vi "Advance Folder Operation.vi"(0 "VISA resource name":refnum<visa-resource-name>, 1 "New File Name":string, 5 "Folder Operation (3: Query Path Type)":i32(ring)=3 items=["Rename File", "Remove File", "Remove Folder", "Query Path Type", "Create New Folder", "List Folder Files"], 7 "File Name":string, 9 "Path (/usb1/)":string="/usb1/", 11 "error in (no error)":errorcluster) -> (3 "Folder File List":string[](array[string]), 4 "VISA resource name out":refnum<visa-resource-name>, 6 "Directory":bool, 8 "File":bool, 10 "Path":string, 15 "error out":errorcluster)   [LabVIEW 2019, in "Keithley 2600 Series.lvlib"]
doc: "Advance operations for the folder and files."
uses:
  Keithley 2600 Series.lvlib
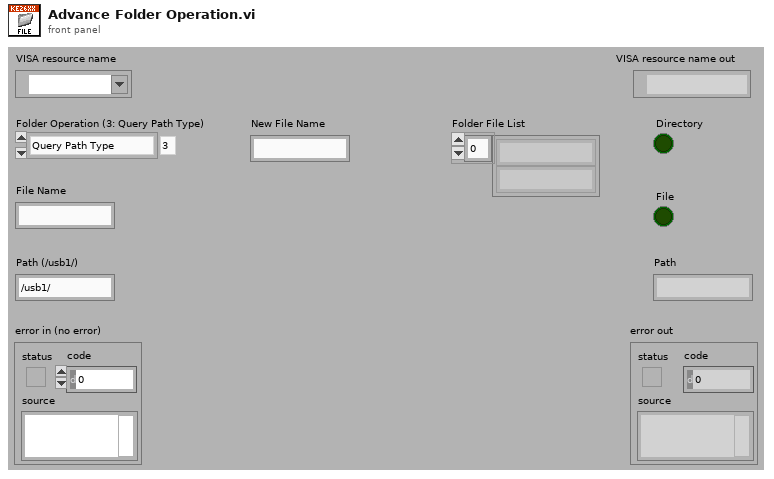
[diagram p1: front panel]
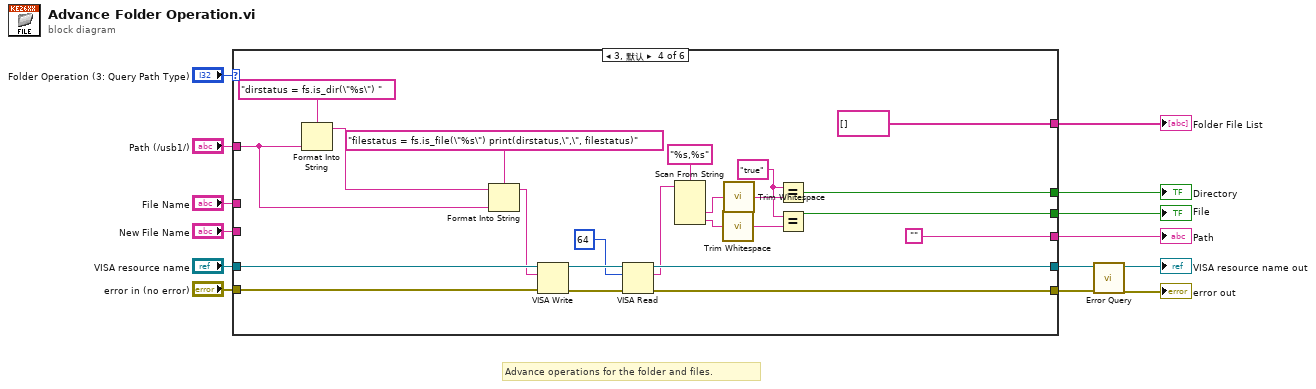
[diagram p0: block diagram]
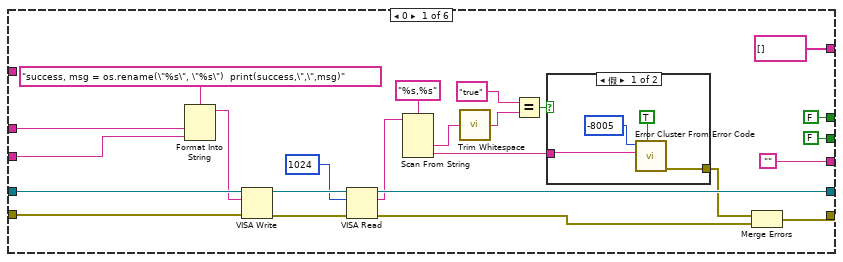
[diagram p2: hidden frame]
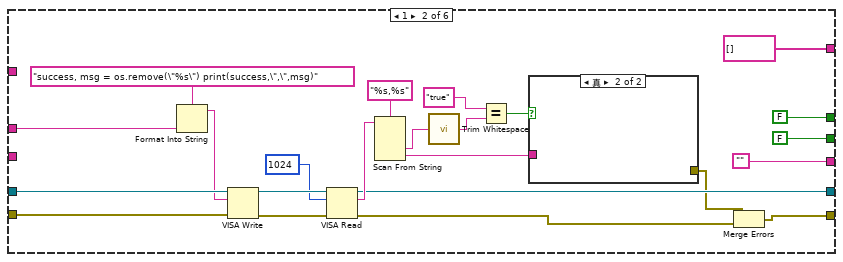
[diagram p4: hidden frame]
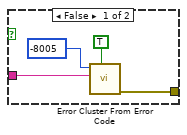
[diagram p5: hidden frame]
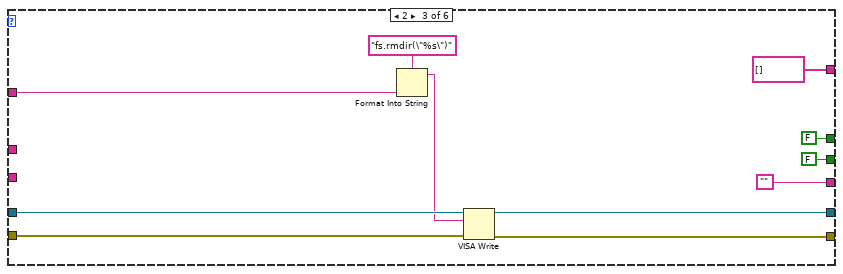
[diagram p6: hidden frame]
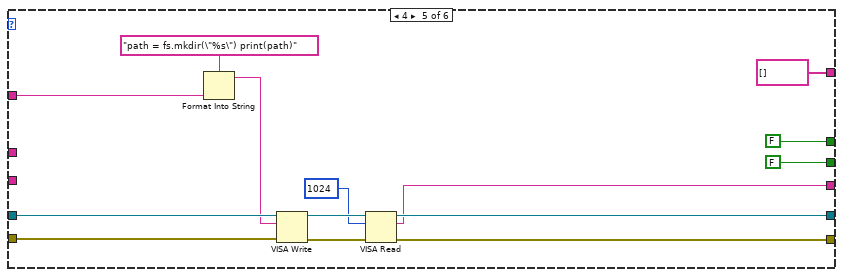
[diagram p7: hidden frame]
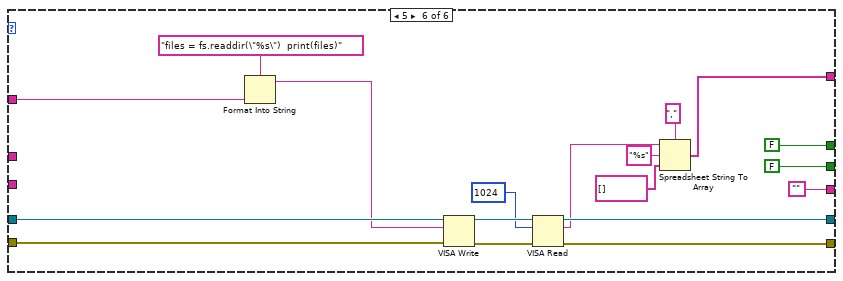
[diagram p8: hidden frame]
diagram:
  # "Advance operations for the folder and files."
  n1 = case shown="3, 默认" "Folder Operation (3: Query Path Type)" {
    tunnel: "VISA resource name" -> [w34 w53 w78 w101 w112 w130]
    tunnel: "error in (no error)" -> [w33 w52 w77 w100 w111 w129]
    tunnel: [w28 w50 w75 w97 w109 w127] -> w4
    tunnel: [w19 w43 w74 w96 w108 w126] -> w3
    tunnel: "Path (/usb1/)" -> [_ _ w79 w95 w113 w131]
    tunnel: "File Name" -> [w32 w64 _ _ _ _]
    tunnel: "New File Name" -> [w31 _ _ _ _ _]
    tunnel: ["" "" "" "" w107 ""] -> w6
    tunnel: [string[] [] string[] [] string[] [] string[] [] string[] [] w122] -> w5
    tunnel: [FALSE FALSE FALSE w82 FALSE FALSE] -> w2
    tunnel: [FALSE FALSE FALSE w81 FALSE FALSE] -> w1
    frame 0 {
      n2 = Format Into String(format string="success, msg = os.rename(\"%s\", \"%s\")  print(success,\",\",msg)", w32, w31) -> (resulting string=w30:string)  [unwired: 2 in, 1 out]
      n3 = VISA Write(VISA resource name=w34, write buffer=w30, error in (no error)=w33) -> (VISA resource name out=w37:refnum<visa-resource-name>, error out=w36:errorcluster)  [unwired: 1 out]
      n4 = VISA Read(VISA resource name=w37, byte count=u32 1024, error in (no error)=w36) -> (VISA resource name out=w28:refnum<visa-resource-name>, read buffer=w27:string, error out=w17:errorcluster)  [unwired: 1 out]
      n5 = Scan From String(format string="%s,%s", input string=w27) -> (output 1=w26:string, output 2=w22:string)  [unwired: 4 in, 3 out]
      n6 = call <vilib>:"Trim Whitespace.vi"("string"=w26) -> ("trimmed string"=w25:string)  [unwired: 1 in]
      n7 = Equal?(x="true", y=w25) -> (x = y?=w23:bool)
      n8 = case shown="假" w23 {
        tunnel: w22 -> [w42 _]
        tunnel: [w40 _] -> w18
        frame False {
          n9 = call <vilib>:"Error Cluster From Error Code.vi"("show call chain? (False)"=TRUE, "error message (\"\")"=w42, "error code (0)"=-8005) -> ("error out"=w40:errorcluster)  [unwired: 6 in]
        }
        frame True {
        }
      }
      n10 = Merge Errors(w18, w17) -> (w19:errorcluster)
    }
    frame 1 {
      n11 = Format Into String(format string="success, msg = os.remove(\"%s\") print(success,\",\",msg)", w64) -> (resulting string=w51:string)  [unwired: 2 in, 1 out]
      n12 = VISA Write(VISA resource name=w53, write buffer=w51, error in (no error)=w52) -> (VISA resource name out=w63:refnum<visa-resource-name>, error out=w62:errorcluster)  [unwired: 1 out]
      n13 = VISA Read(VISA resource name=w63, byte count=u32 1024, error in (no error)=w62) -> (VISA resource name out=w50:refnum<visa-resource-name>, read buffer=w59:string, error out=w46:errorcluster)  [unwired: 1 out]
      n14 = Scan From String(format string="%s,%s", input string=w59) -> (output 1=w58:string, output 2=w54:string)  [unwired: 4 in, 3 out]
      n15 = call <vilib>:"Trim Whitespace.vi"("string"=w58) -> ("trimmed string"=w57:string)  [unwired: 1 in]
      n16 = Equal?(x="true", y=w57) -> (x = y?=w55:bool)
      n17 = case shown="真" w55 {
        tunnel: w54 -> [w69 _]
        tunnel: [w67 _] -> w47
        frame False {
          n18 = call <vilib>:"Error Cluster From Error Code.vi"("show call chain? (False)"=TRUE, "error message (\"\")"=w69, "error code (0)"=-8005) -> ("error out"=w67:errorcluster)  [unwired: 6 in]
        }
        frame True {
        }
      }
      n19 = Merge Errors(w47, w46) -> (w43:errorcluster)
    }
    frame 2 {
      n20 = Format Into String(format string="fs.rmdir(\"%s\")", w79) -> (resulting string=w76:string)  [unwired: 2 in, 1 out]
      n21 = VISA Write(VISA resource name=w78, write buffer=w76, error in (no error)=w77) -> (VISA resource name out=w75:refnum<visa-resource-name>, error out=w74:errorcluster)  [unwired: 1 out]
    }
    frame 3, Default {
      w85 = "true"
      n22 = Format Into String(format string="dirstatus = fs.is_dir(\"%s\") ", w95) -> (resulting string=w94:string)  [unwired: 2 in, 1 out]
      n23 = Format Into String(format string="filestatus = fs.is_file(\"%s\") print(dirstatus,\",\", filestatus)", initial string=w94, w95) -> (resulting string=w93:string)  [unwired: 1 in, 1 out]
      n24 = VISA Write(VISA resource name=w101, write buffer=w93, error in (no error)=w100) -> (VISA resource name out=w99:refnum<visa-resource-name>, error out=w98:errorcluster)  [unwired: 1 out]
      n25 = VISA Read(VISA resource name=w99, byte count=u32 64, error in (no error)=w98) -> (VISA resource name out=w97:refnum<visa-resource-name>, read buffer=w91:string, error out=w96:errorcluster)  [unwired: 1 out]
      n26 = Scan From String(format string="%s,%s", input string=w91) -> (output 1=w89:string, output 2=w88:string)  [unwired: 4 in, 3 out]
      n27 = call <vilib>:"Trim Whitespace.vi"("string"=w88) -> ("trimmed string"=w86:string)  [unwired: 1 in]
      n28 = call <vilib>:"Trim Whitespace.vi"("string"=w89) -> ("trimmed string"=w87:string)  [unwired: 1 in]
      n29 = Equal?(x=w85, y=w87) -> (x = y?=w82:bool)
      n30 = Equal?(x=w85, y=w86) -> (x = y?=w81:bool)
    }
    frame 4 {
      n31 = Format Into String(format string="path = fs.mkdir(\"%s\") print(path)", w113) -> (resulting string=w110:string)  [unwired: 2 in, 1 out]
      n32 = VISA Write(VISA resource name=w112, write buffer=w110, error in (no error)=w111) -> (VISA resource name out=w116:refnum<visa-resource-name>, error out=w115:errorcluster)  [unwired: 1 out]
      n33 = VISA Read(VISA resource name=w116, byte count=u32 1024, error in (no error)=w115) -> (VISA resource name out=w109:refnum<visa-resource-name>, read buffer=w107:string, error out=w108:errorcluster)  [unwired: 1 out]
    }
    frame 5 {
      n34 = Format Into String(format string="files = fs.readdir(\"%s\")  print(files)", w131) -> (resulting string=w128:string)  [unwired: 2 in, 1 out]
      n35 = VISA Write(VISA resource name=w130, write buffer=w128, error in (no error)=w129) -> (VISA resource name out=w134:refnum<visa-resource-name>, error out=w133:errorcluster)  [unwired: 1 out]
      n36 = VISA Read(VISA resource name=w134, byte count=u32 1024, error in (no error)=w133) -> (VISA resource name out=w127:refnum<visa-resource-name>, read buffer=w125:string, error out=w126:errorcluster)  [unwired: 1 out]
      n37 = Spreadsheet String To Array(delimiter (Tab)=",", format string=w125, spreadsheet string="%s", array type (2D Dbl)=string[] []) -> (array=w122:string[])
    }
  }
  "Directory" <- w2
  "Folder File List" <- w5
  "Path" <- w6
  "File" <- w1
  n38 = call "Error Query.vi"("error in (no error)"=w3, "VISA resource name"=w4) -> ("error out"=→"error out":errorcluster, "VISA resource name out"=→"VISA resource name out":refnum<visa-resource-name>)  [unwired: 6 in, 2 out]
